vi "Telescope Generate HK List.vi"() -> (2 "Channel Names":string[](array[string])=["Telescope RA", "Telescope DEC", "Telescope Moving?", "Telescope Status"], 3 "Channel List":refnum<class "HK Item.lvclass">[](array[class]))   [LabVIEW 2024, in "Telescope.lvclass"]
uses:
  Telescope.lvclass
  hk-channel-class/hk-channel-class/HK Item/HK Item.lvclass
  Telescope cluster Status.ctl
  typedefs/CC cluster RA and DEC.ctl
  Telescope enum Status.ctl
  hk-channel-class/hk-channel-class/HK Item/HK Channel Units and Setup.ctl
  hk-channel-class/hk-channel-class/HK Item/HK Channel enum Data Type.ctl
panel:
  out "Unaccounted for":string[](array[string])
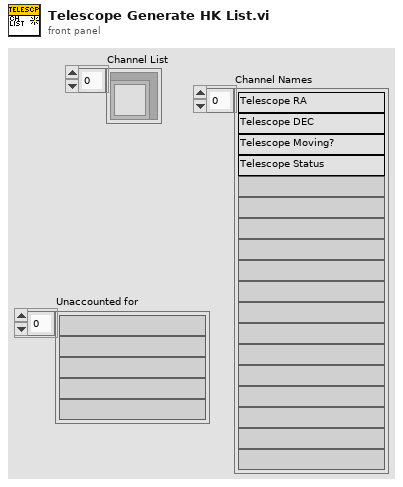
[diagram p1: front panel]
types:
  T1 = typedef "HK Item.lvclass/HK Channel Units and Setup.ctl" = cluster{"Unit Type":string, "Units":string, "Configuration":string, "Digits":i32, "Data Type":T2, "Exponential?":bool, "Source":string}
  T2 = typedef "HK Item.lvclass/HK Channel enum Data Type.ctl" = enum16{"Floating Point", "Integer", "Enum", "String", "Waveform", "File"}
  T3 = typedef "Telescope.lvclass/Telescope cluster Status.ctl" = cluster{"Position":T4, "Connected":bool, "Status":T5, "Curr Time":timestamp, "Status Word":u32, "Focus Pos A":dbl, "UTC Time":timestamp, "Local Sidreal Time":dbl, "Azimuth":dbl, "Altitude":dbl, "Rotator Angle":dbl, "RA String":string, "DEC String":string, "secZ":dbl, "Focus Pos B":dbl, "Focus Pos A-B":dbl, "Rotator Offset":dbl, "Time Offset":dbl, "Dome Angle":dbl, "Dome Status Word":u32, "Dome Moving":bool}
  T4 = typedef "CC cluster RA and DEC.ctl" = cluster{"RA":dbl, "DEC":dbl}
  T5 = typedef "Telescope.lvclass/Telescope enum Status.ctl" = enum16{"Initializing", "Ready", "Moving", "Focusing", "Error"}
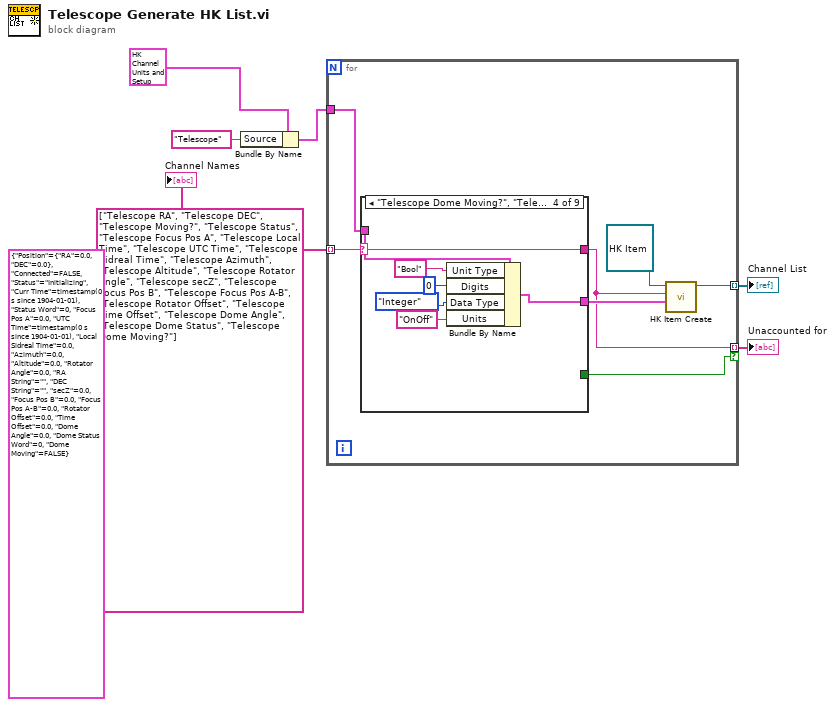
[diagram p0: block diagram]
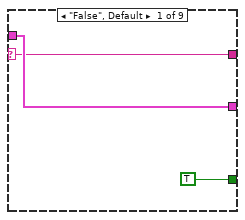
[diagram p2: hidden frame]
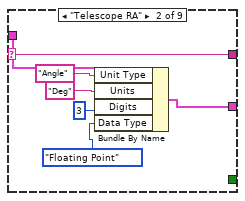
[diagram p3: hidden frame]
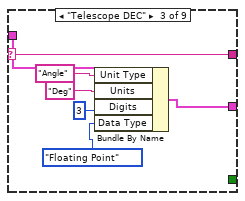
[diagram p4: hidden frame]
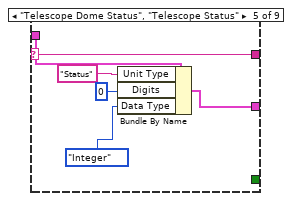
[diagram p5: hidden frame]
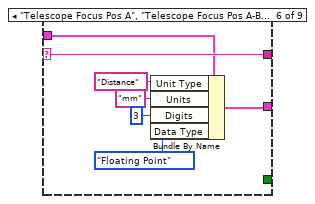
[diagram p6: hidden frame]
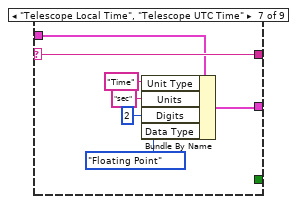
[diagram p7: hidden frame]
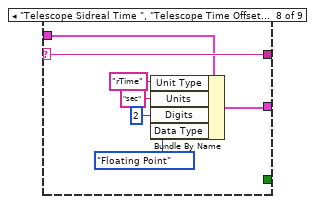
[diagram p8: hidden frame]
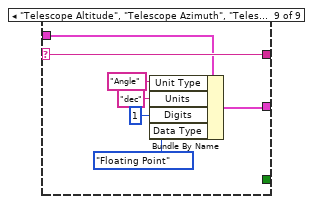
[diagram p9: hidden frame]
diagram:
  (unwired) T3 {"Position"={"RA"=0.0, "DEC"=0.0}, "Connected"=FALSE, "Status"=enum."Initializing", "Curr Time"=timestamp(0 s since 1904-01-01), "Status Word"=0, "Focus Pos A"=0.0, "UTC Time"=timestamp(0 s since 1904-01-01), "Local Sidreal Time"=0.0, "Azimuth"=0.0, "Altitude"=0.0, "Rotator Angle"=0.0, "RA String"="", "DEC String"="", "secZ"=0.0, "Focus Pos B"=0.0, "Focus Pos A-B"=0.0, "Rotator Offset"=0.0, "Time Offset"=0.0, "Dome Angle"=0.0, "Dome Status Word"=0, "Dome Moving"=FALSE} ("Telescope Status")
  w6 = string[] ["Telescope RA", "Telescope DEC", "Telescope Moving?", "Telescope Status", "Telescope Focus Pos A", "Telescope Local Time", "Telescope UTC Time", "Telescope Sidreal Time", "Telescope Azimuth", "Telescope Altitude", "Telescope Rotator Angle", "Telescope secZ", "Telescope Focus Pos B", "Telescope Focus Pos A-B", "Telescope Rotator Offset", "Telescope Time Offset", "Telescope Dome Angle", "Telescope Dome Status", "Telescope Dome Moving?"]
  n1 = Bundle By Name(cluster=T1 {"Unit Type"="", "Units"="", "Configuration"="", "Digits"=3, "Data Type"=enum."Floating Point", "Exponential?"=FALSE, "Source"=""} ("Channel Setup"), "Source"="Telescope") -> (w2:T1)
  n2 = for {
    tunnel: w6 -> [w13] mode=indexing
    tunnel: [w10] -> w5 mode=indexing
    tunnel: [w8] -> w4 mode=indexing if=w9
    tunnel: w2 -> [w7]
    n3 = case shown="\"Telescope Dome Moving?\", \"Telescope Moving?\"" w13 {
      selector: w13 -> [w15 w17 w24 w32 w38 w50 w57 w64 w71]
      tunnel: w7 -> [w16 w23 w30 w37 w43 w49 w56 w63 w70]
      tunnel: [w16 w18 w25 w33 w39 w44 w51 w58 w65] -> w12
      tunnel: [w15 w17 w24 w32 w38 w50 w57 w64 w71] -> w8
      tunnel: [TRUE _ _ _ _ _ _ _ _] -> w9
      frame "False", Default {
      }
      frame "Telescope RA" {
        n4 = Bundle By Name(cluster=w23, "Unit Type"="Angle", "Units"="Deg", "Digits"=3, "Data Type"=HK_Channel_enum_Data_Type."Floating Point") -> (w18:T1)
      }
      frame "Telescope DEC" {
        n5 = Bundle By Name(cluster=w30, "Unit Type"="Angle", "Units"="Deg", "Digits"=3, "Data Type"=HK_Channel_enum_Data_Type."Floating Point") -> (w25:T1)
      }
      frame "Telescope Dome Moving?", "Telescope Moving?" {
        n6 = Bundle By Name(cluster=w37, "Unit Type"="Bool", "Digits"=0, "Data Type"=HK_Channel_enum_Data_Type."Integer", "Units"="OnOff") -> (w33:T1)
      }
      frame "Telescope Dome Status", "Telescope Status" {
        n7 = Bundle By Name(cluster=w43, "Unit Type"="Status", "Digits"=0, "Data Type"=HK_Channel_enum_Data_Type."Integer") -> (w39:T1)
      }
      frame "Telescope Focus Pos A", "Telescope Focus Pos A-B", "Telescope Focus Pos B" {
        n8 = Bundle By Name(cluster=w49, "Unit Type"="Distance", "Units"="mm" ("Unit Type"), "Digits"=3, "Data Type"=HK_Channel_enum_Data_Type."Floating Point") -> (w44:T1)
      }
      frame "Telescope Local Time", "Telescope UTC Time" {
        n9 = Bundle By Name(cluster=w56, "Unit Type"="Time", "Units"="sec" ("Unit Type"), "Digits"=2, "Data Type"=HK_Channel_enum_Data_Type."Floating Point") -> (w51:T1)
      }
      frame "Telescope Sidreal Time ", "Telescope Time Offset" {
        n10 = Bundle By Name(cluster=w63, "Unit Type"="rTime", "Units"="sec" ("Unit Type"), "Digits"=2, "Data Type"=HK_Channel_enum_Data_Type."Floating Point") -> (w58:T1)
      }
      frame "Telescope Altitude", "Telescope Azimuth", "Telescope Dome Angle", "Telescope Rotator Angle", "Telescope Rotator Offset", "Telescope secZ" {
        n11 = Bundle By Name(cluster=w70, "Unit Type"="Angle", "Units"="dec" ("Unit Type"), "Digits"=1, "Data Type"=HK_Channel_enum_Data_Type."Floating Point") -> (w65:T1)
      }
    }
    n12 = call-dynamic "HK Item Create.vi"("Channel Setup"=w12, "Name"=w8, "HK Item in"=refnum<class "HK Item.lvclass"> refnum) -> ("HK Item out"=w10:refnum<class "HK Item.lvclass">)  [unwired: 7 in, 1 out]
  }
  "Channel List" <- w5
  "Unaccounted for" <- w4
  "Channel Names" <- w6
